vi "MFLI module main.vi"(8 "Update timer[ms]":u32=100, 9 "Master mailbox":T6, 11 "Module mailbox":T6) -> ()   [LabVIEW 2024, in "Lock-in module.lvlib"]
doc: "Module to control MFLI form ZhInst.\nKey typedefs: MFLI_message for module, MFLI_command enum [Initialize, Update, Set module, Set Individual parameters, Set parametres, Get point, Get array, Disconnect, End], MFLI_parameter and value{MFLI_node, value}"
uses:
  Lock-in module.lvlib
  Messenger service/Data types/Mailbox address.ctl
  ctl/ACQ status.ctl
  <instrlib>/Zurich Instruments LabOne/Public/ziTypeHandle.ctl
  <instrlib>/Zurich Instruments LabOne/Public/Modules/ziTypeModHandle.ctl
  ctl/ACQ info.ctl
  ctl/Mode.ctl
  Messenger service/Data types/Module name.ctl
  ctl/MFLI_message for module.ctl
  ctl/MFLI_command enum.ctl
  ctl/MFLI parameters.ctl
  <instrlib>/Zurich Instruments LabOne/Public/Modules/ziTypeModEnum.ctl
  ctl/MFLI_parameter and value.ctl
  ctl/MFLI_node.ctl
  <instrlib>/Zurich Instruments LabOne/Public/Configure/ziSetValueDoubleArray.vi
  <instrlib>/Zurich Instruments LabOne/Public/Configure/ziSetValueDouble.vi
  <instrlib>/Zurich Instruments LabOne/Zurich Instruments LabOne.lvlib
  Messenger service/MessengerLib.lvlib
panel:
  out "error IO":errorcluster
  out "Modulation amplitude [A]":dbl
  out "Multimeter name":string
  out "Multimeter port":refnum<visa-resource-name>
  out "Mode":T1=enum."Point"
  out "ACQ  status":T2={"Lock-in Handle"={"handleValid"=FALSE, "Conn"=0, "Path Prefix"="", "Handle"=0, "Connected"=FALSE, "Clockbase(s)"=0.0}, "Address"="DEV", "ModuleHandles"=[], "Lock-in info"={"In50"=FALSE, "InAC"=FALSE, "InDiff"=FALSE, "Out50"=FALSE, "OutEN"=FALSE, "OutF[Hz]"=0.0, "OutA[V]"=0.0, "DemEN"=FALSE, "Const[ms]"=0.0, "Order[-]"=0, "Phase [°]"=0.0}} {"ModuleHandles"."ModHandle" format="0x%08x"; "ModuleHandles"."Conn" format="0x%08x"; "Lock-in Handle"."Handle" format="0x%08x"; "Lock-in Handle"."Conn" format="0x%08x"}
  out "Selected Device":string
  out "Ended":bool
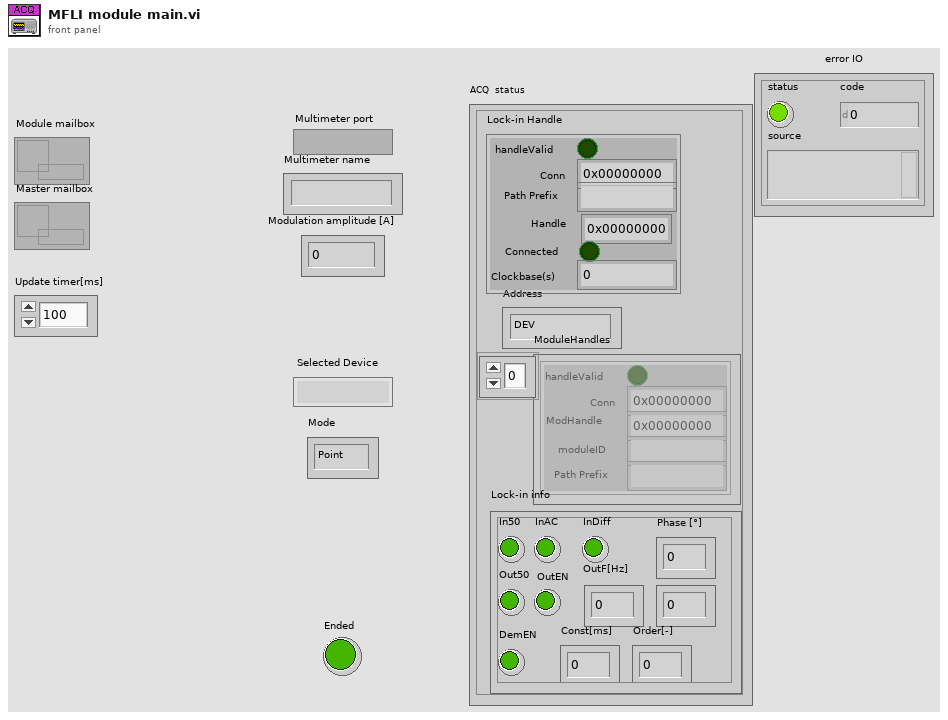
[diagram p1: front panel]
types:
  T1 = typedef "Lock-in module.lvlib/Mode.ctl" = enum16{"None", "Point", "Scope", "Both", "DAQ"}
  T2 = typedef "Lock-in module.lvlib/ACQ status.ctl" = cluster{"Lock-in Handle":T3, "Address":string, "ModuleHandles":T4[], "Lock-in info":T5}
  T3 = typedef "Zurich Instruments LabOne.lvlib/ziTypeHandle.ctl" = cluster{"handleValid":bool, "Conn":u64, "Path Prefix":string, "Handle":u64, "Connected":bool, "Clockbase(s)":dbl}
  T4 = typedef "Zurich Instruments LabOne.lvlib/ziTypeModHandle.ctl" = cluster{"handleValid":bool, "Conn":u64, "ModHandle":u64, "moduleID":string, "Path Prefix":string}
  T5 = typedef "Lock-in module.lvlib/ACQ info.ctl" = cluster{"In50":bool, "InAC":bool, "InDiff":bool, "Out50":bool, "OutEN":bool, "OutF[Hz]":dbl, "OutA[V]":dbl, "DemEN":bool, "Const[ms]":dbl, "Order[-]":i32, "Phase [°]":dbl}
  T6 = typedef "MessengerLib.lvlib/Mailbox address.ctl" = refnum<queue>
  T7 = typedef "Lock-in module.lvlib/MFLI_message for module.ctl" = cluster{"Command":T8, "Data":variant}
  T8 = typedef "Lock-in module.lvlib/MFLI_command enum.ctl" = enum16{"Initialize", "Update", "Set parameters", "Set module", "Set individual parameters", "Get point", "Get array", "Disconnect", "End", "Ignore"}
  T9 = typedef "Module name.ctl" = enum16{"Emty", "Magnet", "VTI", "Excitation", "Servo", "Acquisition", "Rotator", "Digitizer", "SMU2450", "Carousel", "Multimeter", "Tmp monitor", "Power monitor"}
  T10 = typedef "Lock-in module.lvlib/MFLI parameters.ctl" = cluster{"Filter order":dbl, "Filter tau [ms]":dbl, "F_Mod [kHz]":dbl, "Amp_Mod [mV]":dbl, "Enable output":u16, "Phase [°]":dbl}
  T11 = typedef "Lock-in module.lvlib/MFLI_parameter and value.ctl" = cluster{"parameter":T12, "value":dbl}
  T12 = typedef "Lock-in module.lvlib/MFLI_node.ctl" = enum16{"None", "filter_order [-]", "filter_constant [ms]", "in_diff", "in_autorange", "in_imp50", "in_AC", "osc_freq [kHz]", "out_ampl [V]", "out_autorange", "out_imp50", "enable output", "enamble ampl", "scope_enable", "scope_rate", "scope_len", "scope_trigEn", "AuxOut_amplify", "Phase_deg", "AuxOut_select"}
  T13 = typedef "Zurich Instruments LabOne.lvlib/ziTypeModEnum.ctl" = u16
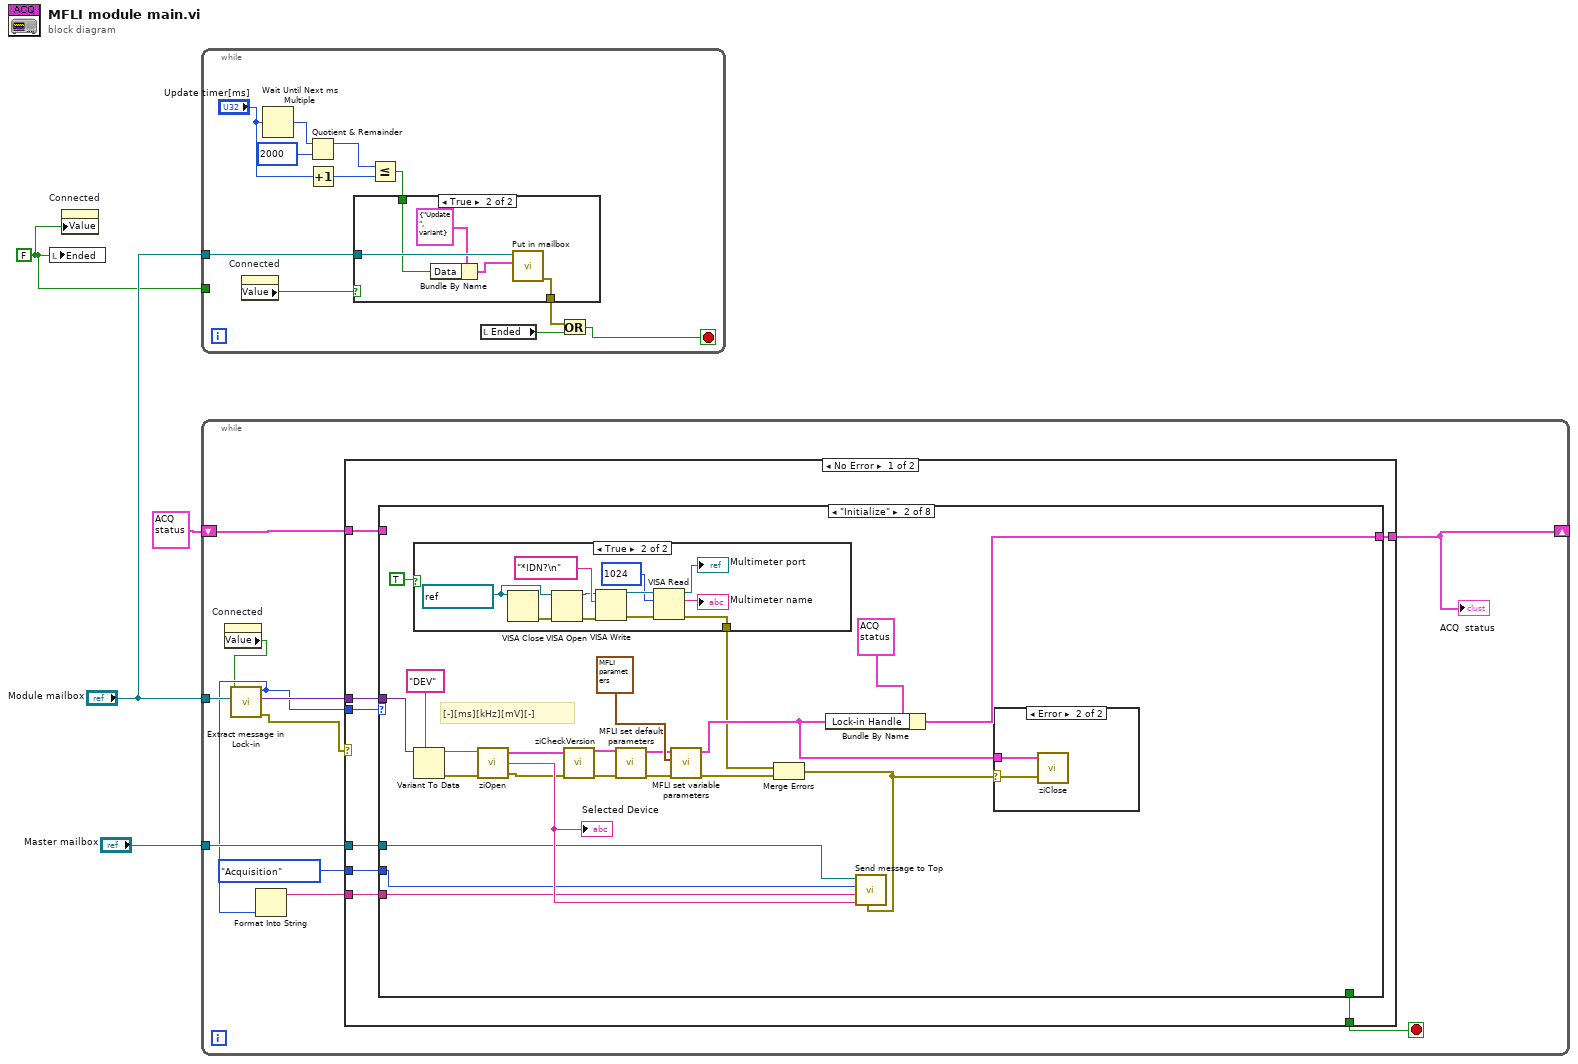
[diagram p0: block diagram]
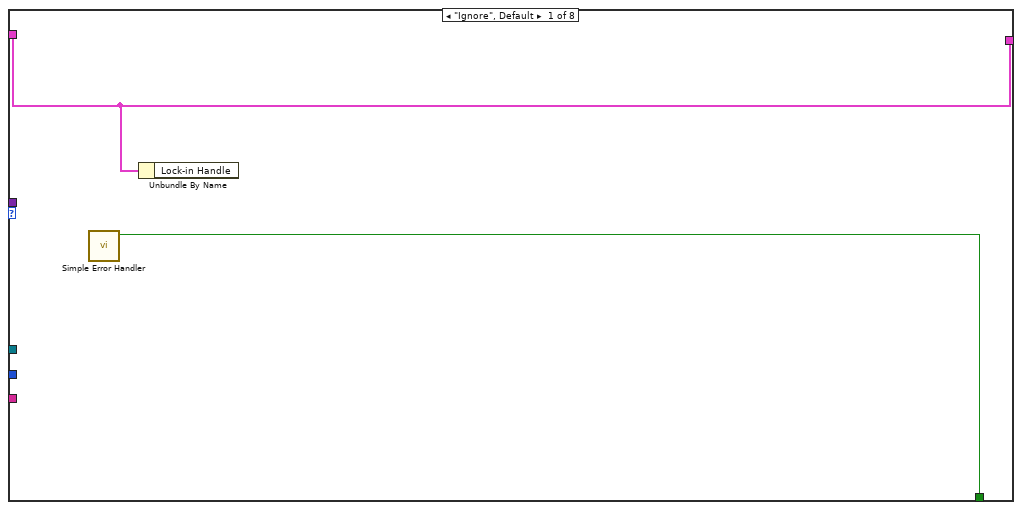
[diagram p2: hidden frame]
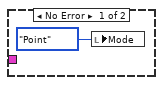
[diagram p4: hidden frame]
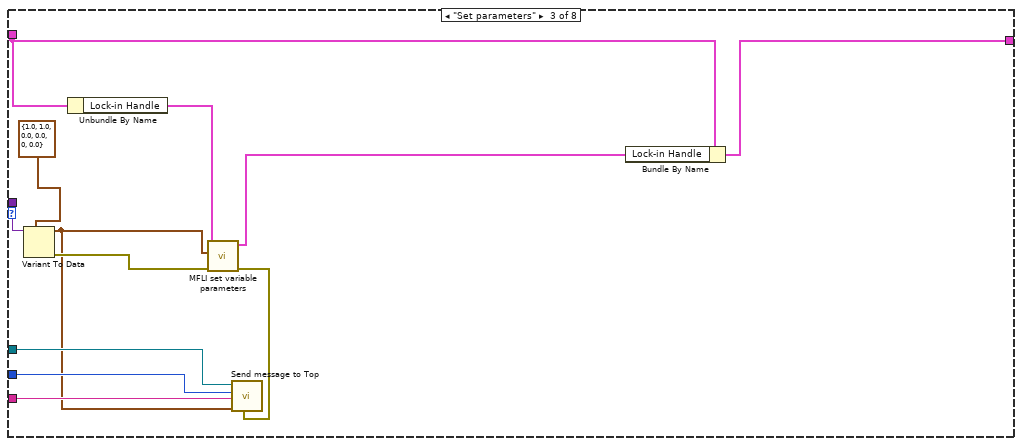
[diagram p5: hidden frame]
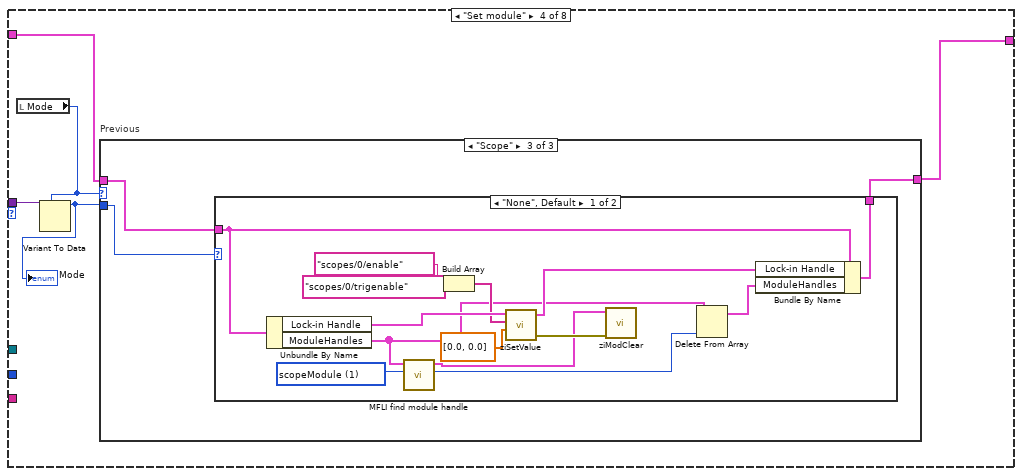
[diagram p6: hidden frame]
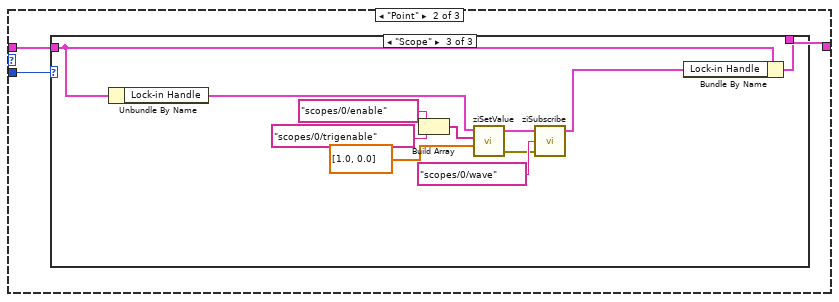
[diagram p8: hidden frame]
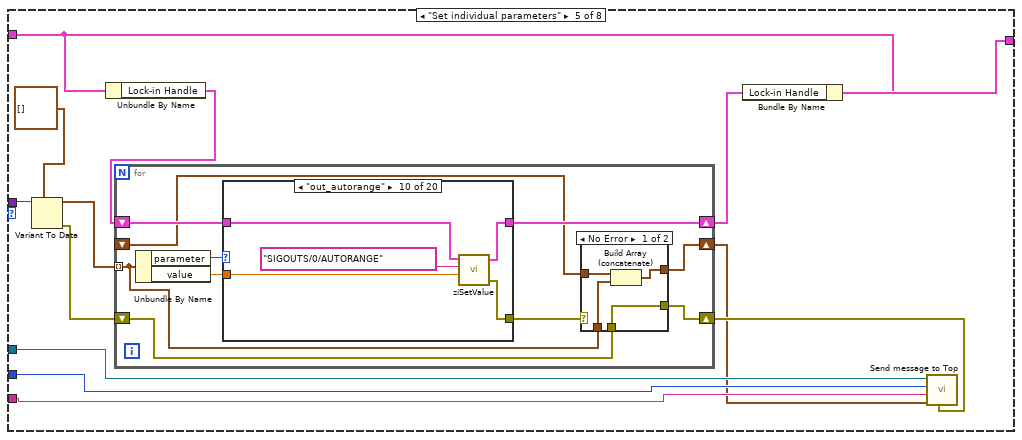
[diagram p12: hidden frame]
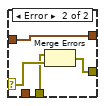
[diagram p13: hidden frame]
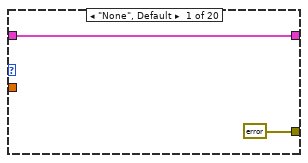
[diagram p14: hidden frame]
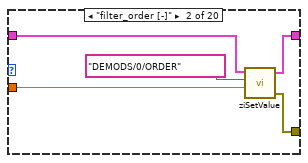
[diagram p15: hidden frame]
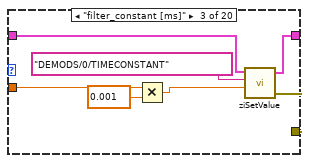
[diagram p16: hidden frame]
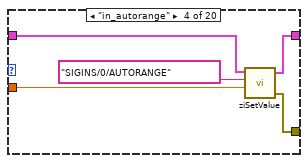
[diagram p17: hidden frame]
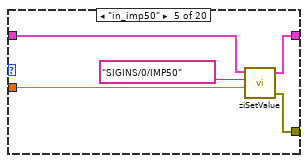
[diagram p18: hidden frame]
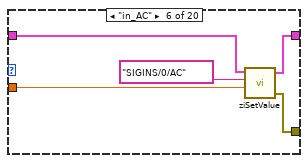
[diagram p19: hidden frame]
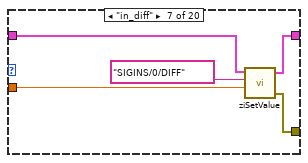
[diagram p20: hidden frame]
diagram:
  w1 = FALSE ("Initialized")
  n1 = local write "Ended"(w1) -> ()
  n2 = property on="Connected" class="Bool (strict)"("Value"=w1) -> ()  [unwired: 2 in, 2 out]
  n3 = while {
    tunnel: "Module mailbox" -> [w15]
    tunnel: w1 -> [_]
    stop <- w6 stop-if-true
    n4 = property on="Connected" class="Bool (strict)"() -> ("Value"=w8:bool)  [unwired: 2 in, 2 out]
    n5 = Wait Until Next ms Multiple(millisecond multiple="Update timer[ms]") -> (millisecond timer value=w14:u32)
    n6 = Quotient & Remainder(x=w14, y=u32 2000) -> (x-y*floor(x/y)=w12:u32)  [unwired: 1 out]
    n7 = Increment(x="Update timer[ms]") -> (x+1=w9:u32)
    n8 = Less Or Equal?(x=w12, y=w9) -> (x <= y?=w10:bool)
    n9 = case shown="True" w8 {
      tunnel: w15 -> [_ w20]
      tunnel: w10 -> [_ w17]
      tunnel: [_ w16] -> w7
      frame False {
      }
      frame True {
        n10 = Bundle By Name(cluster=T7 {"Command"=enum."Update", "Data"=variant} ("MSG for  ACQ"), "Data"=w17) -> (w18:T7)
        n11 = call "Put in mailbox.vi"("Message"=w18, "Queue in"=w20) -> ("error out"=w16:errorcluster)  [unwired: 7 in, 2 out]
      }
    }
    n12 = local read "Ended"() -> (w5:bool)
    n13 = Or(x=w7, y=w5) -> (x .or. y?=w6:bool)
  }
  n14 = while {
    tunnel: "Module mailbox" -> [w31]
    tunnel: "Master mailbox" -> [w30]
    shift-right: [w24] -> _
    shift-left: T2 {"Lock-in Handle"={"handleValid"=FALSE, "Conn"=0, "Path Prefix"="", "Handle"=0, "Connected"=FALSE, "Clockbase(s)"=0.0}, "Address"="DEV", "ModuleHandles"=[], "Lock-in info"={"In50"=FALSE, "InAC"=FALSE, "InDiff"=FALSE, "Out50"=FALSE, "OutEN"=FALSE, "OutF[Hz]"=0.0, "OutA[V]"=0.0, "DemEN"=FALSE, "Const[ms]"=0.0, "Order[-]"=0, "Phase [°]"=0.0}} -> [w28]
    stop <- w23 stop-if-true
    n15 = property on="Connected" class="Bool (strict)"() -> ("Value"=w22:bool)  [unwired: 2 in, 2 out]
    n16 = call "Extract message in Lock-in.vi"("Module mailbox"=w31, "Initialized?"=w22) -> ("error out"=w21:errorcluster, "Data"=w29:variant, "Command out"=w25:T8)  [unwired: 7 in]
    n17 = Format Into String(w25) -> (resulting string=w27:string)  [unwired: 3 in, 1 out]
    n18 = case shown="No Error" w21 {
      selector: w21 -> [_ w345]
      tunnel: w30 -> [w39 _]
      tunnel: w29 -> [w38 _]
      tunnel: w28 -> [w37 w344]
      tunnel: w27 -> [w36 _]
      tunnel: Module_name."Acquisition" ("Module") -> [w35 _]
      tunnel: w25 -> [w34 _]
      tunnel: [w33 w344] -> w24
      tunnel: [w32 w346] -> w23
      frame No Error {
        n19 = case shown="\"Initialize\"" w34 {
          tunnel: w39 -> [_ w57 w85 _ w133 w278 w319 w336]
          tunnel: w38 -> [_ w63 w89 w94 w142 w273 _ _]
          tunnel: [w41 _ _ _ _ _ w310 FALSE] -> w32
          tunnel: [w40 w56 w86 w91 w140 w280 w312 w328] -> w33
          tunnel: w37 -> [w40 _ w87 w90 w138 w277 w320 w337]
          tunnel: w36 -> [_ w53 w84 _ w135 w276 w317 w333]
          tunnel: w35 -> [_ w52 w83 _ w134 w265 w318 w334]
          frame "Ignore", Default {
            n20 = call <vilib>:"Simple Error Handler.vi"() -> ("error?"=w41:bool)  [unwired: 5 in, 4 out]
            n21 = Unbundle By Name(w40) -> ()  [unwired: 1 out]
          }
          frame "Initialize" {
            # "[-][ms][kHz][mV][-]"
            n22 = case shown="True" TRUE {
              tunnel: [_ w66] -> w43
              frame False {
              }
              frame True {
                w73 = refnum<visa-resource-name> "COM6" ("VISA resource name")
                n23 = VISA Close(VISA resource name=w73) -> (error out=w74:errorcluster)  [unwired: 1 in]
                n24 = VISA Open(error in (no error)=w74, VISA resource name=w73) -> (VISA resource name=w68:refnum<visa-resource-name>, error out=w67:errorcluster)  [unwired: 3 in]
                n25 = VISA Write(VISA resource name=w68, write buffer="*IDN?\n", error in (no error)=w67) -> (VISA resource name out=w72:refnum<visa-resource-name>, error out=w71:errorcluster)  [unwired: 1 out]
                n26 = VISA Read(VISA resource name=w72, byte count=u32 1024, error in (no error)=w71) -> (VISA resource name out=→"Multimeter port":refnum<visa-resource-name>, read buffer=→"Multimeter name":string, error out=w66:errorcluster)  [unwired: 1 out]
              }
            }
            n27 = Variant To Data(type="DEV" ("Address"), Variant=w63) -> (data=w61:string, error out=w60:errorcluster)  [unwired: 1 in]
            n28 = call <instrlib>:"ziOpen.vi"("Error In"=w60, "Address"=w61) -> ("Error Out"=w54:errorcluster, "Selected Device"=w58:string, "HandleOut"=w55:T3)  [unwired: 2 in]
            "Selected Device" <- w58
            n29 = call <instrlib>:"ziCheckVersion.vi"("Handle In"=w55, "Error In"=w54) -> ("Handle Out"=w50:T3, "Error Out"=w51:errorcluster)  [unwired: 11 in, 1 out]
            n30 = call "MFLI set default parameters.vi"("error in (no error)"=w51, "Lock-in Handle"=w50) -> ("Error Out"=w47:errorcluster, "Handle Out"=w48:T3)  [unwired: 8 in]
            n31 = call "MFLI set variable parameters.vi"("error in"=w47, "ACQ parameters"=T10 {"Filter order"=5.0, "Filter tau [ms]"=50.0, "F_Mod [kHz]"=10.0, "Amp_Mod [mV]"=100.0, "Enable output"=0, "Phase [°]"=0.0}, "handle in"=w48) -> ("Error Out"=w46:errorcluster, "Handle Out"=w44:T3)  [unwired: 7 in]
            n32 = Merge Errors(w43, w46) -> (w45:errorcluster)
            n33 = Bundle By Name(cluster=T2 {"Lock-in Handle"={"handleValid"=FALSE, "Conn"=0, "Path Prefix"="", "Handle"=0, "Connected"=FALSE, "Clockbase(s)"=0.0}, "Address"="DEV", "ModuleHandles"=[], "Lock-in info"={"In50"=FALSE, "InAC"=FALSE, "InDiff"=FALSE, "Out50"=FALSE, "OutEN"=FALSE, "OutF[Hz]"=0.0, "OutA[V]"=0.0, "DemEN"=FALSE, "Const[ms]"=0.0, "Order[-]"=0, "Phase [°]"=0.0}}, "Lock-in Handle"=w44) -> (w56:T2)
            n34 = call "Send message to Top.vi"("Error in (no error)"=w45, "Data"=w58, "Response"=w53, "Module"=w52, "Mailbox address in"=w57) -> ()  [unwired: 5 in, 2 out]
            n35 = case shown="Error" w45 {
              selector: w45 -> [_ w77]
              tunnel: w44 -> [_ w76]
              frame No Error {
                n36 = local write "Mode"(Mode."Point" ("Mode")) -> ()
              }
              frame Error {
                n37 = call <instrlib>:"ziClose.vi"("Error In"=w77, "Handle In"=w76) -> ()  [unwired: 2 in, 2 out]
              }
            }
          }
          frame "Set parameters" {
            n38 = Variant To Data(type=T10 {"Filter order"=1.0, "Filter tau [ms]"=1.0, "F_Mod [kHz]"=0.0, "Amp_Mod [mV]"=0.0, "Enable output"=0, "Phase [°]"=0.0} ("ACQ parameters"), Variant=w89) -> (data=w78:T10, error out=w80:errorcluster)  [unwired: 1 in]
            n39 = Unbundle By Name(w87) -> ("Lock-in Handle"=w81:T3)
            n40 = call "MFLI set variable parameters.vi"("error in"=w80, "ACQ parameters"=w78, "handle in"=w81) -> ("Error Out"=w82:errorcluster, "Handle Out"=w79:T3)  [unwired: 7 in]
            n41 = call "Send message to Top.vi"("Error in (no error)"=w82, "Data"=w78, "Response"=w84, "Module"=w83, "Mailbox address in"=w85) -> ()  [unwired: 5 in, 2 out]
            n42 = Bundle By Name(cluster=w87, "Lock-in Handle"=w79) -> (w86:T2)
          }
          frame "Set module" {
            n43 = local read "Mode"() -> (w93:T1)
            n44 = Variant To Data(type=w93, Variant=w94) -> (data=w92:T1)  [unwired: 1 in, 1 out]
            "Mode" <- w92
            n45 = case "Previous" shown="\"Scope\"" w93 {
              tunnel: w92 -> [_ w98 w114]
              tunnel: w90 -> [w95 w97 w113]
              tunnel: [w95 w96 w112] -> w91
              frame "None", Default {
              }
              frame "Point" {
                n46 = case shown="\"Scope\"" w98 {
                  tunnel: w97 -> [w99 w100 w110]
                  tunnel: [w99 w100 w111] -> w96
                  frame "None", Default {
                  }
                  frame "Point" {
                  }
                  frame "Scope" {
                    n47 = Unbundle By Name(w110) -> ("Lock-in Handle"=w101:T3)
                    n48 = Build Array("scopes/0/enable", "scopes/0/trigenable") -> (w107:string[])
                    n49 = call-poly <instrlib>:"ziSetValue.vi"("Values"=dbl[] [1.0, 0.0] ("Value"), "Paths"=w107, "Handle In"=w101) -> ("Error Out"=w102:errorcluster, "Handle Out"=w104:T3)  [unwired: 2 in]
                    n50 = call <instrlib>:"ziSubscribe.vi"("error in"=w102, "Path ()"="scopes/0/wave" ("Path"), "Handle In"=w104) -> ("Handle Out"=w103:T3)  [unwired: 1 in, 1 out]
                    n51 = Bundle By Name(cluster=w110, "Lock-in Handle"=w103) -> (w111:T2)
                  }
                }
              }
              frame "Scope" {
                n52 = case shown="\"None\", Default" w114 {
                  tunnel: [w128 w129] -> w112
                  tunnel: w113 -> [w119 w129]
                  frame "None", Default {
                    w120 = T13 1 items=["sweep", "scopeModule", "dataAcquisitionModule", "pidAdvisor", "awgModule", "impedanceModule", "multiDeviceSyncModule", "zoomFFT", "trigger", "deviceSettings", "record"] ("module Id")
                    n53 = Unbundle By Name(w119) -> ("Lock-in Handle"=w125:T3, "ModuleHandles"=w116:T4[])
                    n54 = call "MFLI find module handle.vi"("module Id"=w120, "ModuleHandles"=w116) -> ("index"=w117:i32, "ziModHandle out"=w118:T4)  [unwired: 7 in, 1 out]
                    n55 = Build Array("scopes/0/enable", "scopes/0/trigenable") -> (w122:string[])
                    n56 = call-poly <instrlib>:"ziSetValue.vi"("Values"=dbl[] [0.0, 0.0] ("Value"), "Paths"=w122, "Handle In"=w125) -> ("Error Out"=w123:errorcluster, "Handle Out"=w124:T3)  [unwired: 2 in]
                    n57 = call <instrlib>:"ziModClear.vi"("Error In"=w123, "ziModHandle In"=w118) -> ()  [unwired: 7 in, 2 out]
                    n58 = Delete From Array(array=w116, index=w117) -> (array with subset deleted=w115:T4[])  [unwired: 1 in, 1 out]
                    n59 = Bundle By Name(cluster=w119, "Lock-in Handle"=w124, "ModuleHandles"=w115) -> (w128:T2)
                  }
                  frame "Scope" {
                  }
                }
              }
            }
          }
          frame "Set individual parameters" {
            n60 = Variant To Data(type=T11[] [] ("Array"), Variant=w142) -> (data=w136:T11[], error out=w131:errorcluster)  [unwired: 1 in]
            n61 = Unbundle By Name(w138) -> ("Lock-in Handle"=w139:T3)
            n62 = for {
              tunnel: w136 -> [w145] mode=indexing
              shift-right: [w151] -> w137
              shift-left: w139 -> [w152]
              shift-right: [w147] -> w132
              shift-left: w131 -> [w146]
              shift-right: [w144] -> w130
              shift-left: _ -> [w143]
              n63 = Unbundle By Name(w145) -> ("parameter"=w149:T12, "value"=w150:dbl)
              n64 = case shown="\"out_autorange\"" w149 {
                tunnel: w152 -> [w162 w167 w174 w179 w184 w189 w194 w201 w206 w211 w216 w221 w226 w231 w234 w241 w244 w249 w254 w259]
                tunnel: [w162 w166 w173 w178 w183 w188 w193 w200 w205 w210 w215 w220 w225 w230 w235 w240 w245 w250 w255 w260] -> w151
                tunnel: w150 -> [_ w165 w172 w177 w182 w187 w192 w197 w204 w209 w214 w219 w224 w228 w233 w239 w243 w248 w253 w258]
                tunnel: [errorcluster {"status"=FALSE, "code"=0, "source"=""} ("Error Out") w163 w170 w175 w180 w185 w190 w199 w202 w207 w212 w217 w222 w229 w236 w237 w246 w251 w256 w261] -> w148
                frame "None", Default {
                }
                frame "filter_order [-]" {
                  n65 = call-poly <instrlib>:"ziSetValue.vi"("Value"=w165, "Path"="DEMODS/0/ORDER", "Handle In"=w167) -> ("Error Out"=w163:errorcluster, "Handle Out"=w166:T3)  [unwired: 2 in]
                }
                frame "filter_constant [ms]" {
                  n66 = Multiply(x=w172, y=0.001) -> (x*y=w169:dbl)
                  n67 = call-poly <instrlib>:"ziSetValue.vi"("Value"=w169, "Path"="DEMODS/0/TIMECONSTANT", "Handle In"=w174) -> ("Error Out"=w170:errorcluster, "Handle Out"=w173:T3)  [unwired: 2 in]
                }
                frame "in_autorange" {
                  n68 = call-poly <instrlib>:"ziSetValue.vi"("Value"=w177, "Path"="SIGINS/0/AUTORANGE", "Handle In"=w179) -> ("Error Out"=w175:errorcluster, "Handle Out"=w178:T3)  [unwired: 2 in]
                }
                frame "in_imp50" {
                  n69 = call-poly <instrlib>:"ziSetValue.vi"("Value"=w182, "Path"="SIGINS/0/IMP50", "Handle In"=w184) -> ("Error Out"=w180:errorcluster, "Handle Out"=w183:T3)  [unwired: 2 in]
                }
                frame "in_AC" {
                  n70 = call-poly <instrlib>:"ziSetValue.vi"("Value"=w187, "Path"="SIGINS/0/AC", "Handle In"=w189) -> ("Error Out"=w185:errorcluster, "Handle Out"=w188:T3)  [unwired: 2 in]
                }
                frame "in_diff" {
                  n71 = call-poly <instrlib>:"ziSetValue.vi"("Value"=w192, "Path"="SIGINS/0/DIFF", "Handle In"=w194) -> ("Error Out"=w190:errorcluster, "Handle Out"=w193:T3)  [unwired: 2 in]
                }
                frame "osc_freq [kHz]" {
                  n72 = Multiply(x=w197, y=1000.0) -> (x*y=w196:dbl)
                  n73 = call-poly <instrlib>:"ziSetValue.vi"("Value"=w196, "Path"="OSCS/0/FREQ", "Handle In"=w201) -> ("Error Out"=w199:errorcluster, "Handle Out"=w200:T3)  [unwired: 2 in]
                }
                frame "out_ampl [V]" {
                  n74 = call-poly <instrlib>:"ziSetValue.vi"("Value"=w204, "Path"="SIGOUTS/0/AMPLITUDES/1", "Handle In"=w206) -> ("Error Out"=w202:errorcluster, "Handle Out"=w205:T3)  [unwired: 2 in]
                }
                frame "out_autorange" {
                  n75 = call-poly <instrlib>:"ziSetValue.vi"("Value"=w209, "Path"="SIGOUTS/0/AUTORANGE", "Handle In"=w211) -> ("Error Out"=w207:errorcluster, "Handle Out"=w210:T3)  [unwired: 2 in]
                }
                frame "out_imp50" {
                  n76 = call-poly <instrlib>:"ziSetValue.vi"("Value"=w214, "Path"="SIGOUTS/0/IMP50", "Handle In"=w216) -> ("Error Out"=w212:errorcluster, "Handle Out"=w215:T3)  [unwired: 2 in]
                }
                frame "enable output" {
                  n77 = call-poly <instrlib>:"ziSetValue.vi"("Value"=w219, "Path"="SIGOUTS/0/ON", "Handle In"=w221) -> ("Error Out"=w217:errorcluster, "Handle Out"=w220:T3)  [unwired: 2 in]
                }
                frame "enamble ampl" {
                  n78 = call-poly <instrlib>:"ziSetValue.vi"("Value"=w224, "Path"="SIGOUTS/0/ENABLES/1", "Handle In"=w226) -> ("Error Out"=w222:errorcluster, "Handle Out"=w225:T3)  [unwired: 2 in]
                }
                frame "scope_enable" {
                  n79 = call-poly <instrlib>:"ziSetValue.vi"("Value"=w228, "Path"="scopes/0/enable", "Handle In"=w231) -> ("Error Out"=w229:errorcluster, "Handle Out"=w230:T3)  [unwired: 2 in]
                }
                frame "scope_rate" {
                  n80 = call-poly <instrlib>:"ziSetValue.vi"("Value"=w233, "Path"="scopes/0/time", "Handle In"=w234) -> ("Error Out"=w236:errorcluster, "Handle Out"=w235:T3)  [unwired: 2 in]
                }
                frame "scope_trigEn" {
                  n81 = call-poly <instrlib>:"ziSetValue.vi"("Value"=w239, "Path"="SCOPES/0/TRIGENABLE", "Handle In"=w241) -> ("Error Out"=w237:errorcluster, "Handle Out"=w240:T3)  [unwired: 2 in]
                }
                frame "scope_len" {
                  n82 = call-poly <instrlib>:"ziSetValue.vi"("Value"=w243, "Path"="scopes/0/length", "Handle In"=w244) -> ("Error Out"=w246:errorcluster, "Handle Out"=w245:T3)  [unwired: 2 in]
                }
                frame "AuxOut_amplify" {
                  n83 = call-poly <instrlib>:"ziSetValue.vi"("Value"=w248, "Path"="auxouts/0/scale", "Handle In"=w249) -> ("Error Out"=w251:errorcluster, "Handle Out"=w250:T3)  [unwired: 2 in]
                }
                frame "Phase_deg" {
                  n84 = call-poly <instrlib>:"ziSetValue.vi"("Value"=w253, "Path"="demods/1/phaseshift", "Handle In"=w254) -> ("Error Out"=w256:errorcluster, "Handle Out"=w255:T3)  [unwired: 2 in]
                }
                frame "AuxOut_select" {
                  n85 = call-poly <instrlib>:"ziSetValue.vi"("Value"=w258, "Path"="auxouts/0/outputselect", "Handle In"=w259) -> ("Error Out"=w261:errorcluster, "Handle Out"=w260:T3)  [unwired: 2 in]
                }
              }
              n86 = case shown="No Error" w148 {
                selector: w148 -> [_ w160]
                tunnel: [w156 w159] -> w147
                tunnel: w146 -> [w156 w158]
                tunnel: w145 -> [w154 _]
                tunnel: [w155 w157] -> w144
                tunnel: w143 -> [w153 w157]
                frame No Error {
                  n87 = Build Array (concatenate)(w153, w154) -> (w155:T11[])
                }
                frame Error {
                  n88 = Merge Errors(w158, w160) -> (w159:errorcluster)
                }
              }
            }
            n89 = Bundle By Name(cluster=w138, "Lock-in Handle"=w137) -> (w140:T2)
            n90 = call "Send message to Top.vi"("Error in (no error)"=w132, "Data"=w130, "Response"=w135, "Module"=w134, "Mailbox address in"=w133) -> ()  [unwired: 5 in, 2 out]
          }
          frame "Update" {
            n91 = Unbundle By Name(w277) -> ("Lock-in info"=w270:T5, "ModuleHandles"=w267:T4[], "Lock-in Handle"=w279:T3)
            n92 = Variant To Data(type=TRUE, Variant=w273) -> (data=w271:bool, error out=w274:errorcluster)  [unwired: 1 in]
            n93 = case shown="True" w271 {
              tunnel: w279 -> [w284 w294]
              tunnel: [w284 w293] -> w266
              tunnel: w278 -> [w281 w292]
              tunnel: [w282 w290] -> w264
              tunnel: w265 -> [_ w289]
              tunnel: [w281 w288] -> w269
              tunnel: w276 -> [_ w287]
              tunnel: [w283 w286] -> w275
              tunnel: w274 -> [w282 w285]
              tunnel: w270 -> [w283 _]
              frame False {
              }
              frame True {
                n94 = call "Lock-in update.vi"("error in (no error)"=w285, "Lock-in Handle"=w294) -> ("error out"=w291:errorcluster, "Lock-in info"=w286:T5, "Handle Out"=w293:T3)  [unwired: 7 in]
                n95 = call "Send message to Top.vi"("Error in (no error)"=w291, "Data"=w286, "Response"=w287, "Module"=w289, "Mailbox address in"=w292) -> ("Error out"=w290:errorcluster, "Mailbox address out"=w288:T6)  [unwired: 5 in]
              }
            }
            n96 = case shown="True" w271 {
              tunnel: w265 -> [_ w300]
              tunnel: w269 -> [_ w297]
              frame False {
              }
              frame True {
                n97 = local read "Multimeter port"() -> (w308:refnum<visa-resource-name>)
                n98 = VISA Write(VISA resource name=w308, write buffer="READ?\n") -> (VISA resource name out=w307:refnum<visa-resource-name>, error out=w296:errorcluster)  [unwired: 1 in, 1 out]
                n99 = VISA Read(VISA resource name=w307, byte count=u32 1024, error in (no error)=w296) -> (read buffer=w305:string, error out=w295:errorcluster)  [unwired: 2 out]
                n100 = String Subset(string=w305, length (rest)=11 ("length (rest)")) -> (substring=w306:string)  [unwired: 1 in]
                n101 = Scan Value(string=w306, format string="%g") -> (value=w299:dbl)  [unwired: 1 in, 1 out]
                "Modulation amplitude [A]" <- w299
                n102 = call "Send message to Top.vi"("Error in (no error)"=w295, "Data"=w299, "Response"="Get ModA", "Module"=w300, "Mailbox address in"=w297) -> ()  [unwired: 5 in, 2 out]
              }
            }
            n103 = local read "Mode"() -> (w268:T1)
            n104 = call "MFLI read data.vi"("Module"=w265, "ModuleHandles in"=w267, "error in (no error)"=w264, "lock-in handle in"=w266, "Mode"=w268, "Queue in"=w269) -> ("ModuleHandles out"=w262:T4[], "Handle Out out"=w263:T3)  [unwired: 4 in]
            n105 = Bundle By Name(cluster=w277, "Lock-in Handle"=w263, "ModuleHandles"=w262, "Lock-in info"=w275) -> (w280:T2)
          }
          frame "End" {
            w310 = TRUE
            n106 = Unbundle By Name(w320) -> ("Lock-in Handle"=w314:T3)
            n107 = local read "Mode"() -> (w316:T1)
            n108 = case shown="\"Scope\", \"Both\"" w316 {
              tunnel: w314 -> [w322 w326]
              tunnel: [w322 w324] -> w315
              tunnel: [_ w323] -> w309
              frame "None", Default {
              }
              frame "Scope", "Both" {
                n109 = call <instrlib>:"ziUnSubscribe.vi"("Path (\"/\")"="scopes/0/wave" ("Path"), "Handle in"=w326) -> ("error out"=w323:errorcluster, "Handle out"=w324:T3)  [unwired: 2 in]
              }
            }
            n110 = call <instrlib>:"ziClose.vi"("Error In"=w309, "Handle In"=w315) -> ("Handle Out"=w311:T3)  [unwired: 2 in, 1 out]
            n111 = call "Send message to Top.vi"("Data"=w311, "Response"=w317, "Module"=w318, "Mailbox address in"=w319) -> ()  [unwired: 6 in, 2 out]
            n112 = case shown="False" TRUE {
              frame False {
              }
              frame True {
                n113 = local read "Multimeter port"() -> (w321:refnum<visa-resource-name>)
                n114 = VISA Close(VISA resource name=w321) -> ()  [unwired: 1 in, 1 out]
              }
            }
            n115 = Bundle By Name(cluster=w320, "Lock-in Handle"=w311) -> (w312:T2)
            "Ended" <- w310
          }
          frame "Disconnect" {
            n116 = Unbundle By Name(w337) -> ("Lock-in Handle"=w330:T3)
            n117 = local read "Mode"() -> (w332:T1)
            n118 = case shown="\"Scope\", \"Both\"" w332 {
              tunnel: w330 -> [w340 w343]
              tunnel: [w340 w341] -> w331
              frame "None", Default {
              }
              frame "Scope", "Both" {
                n119 = call <instrlib>:"ziUnSubscribe.vi"("Path (\"/\")"="scopes/0/wave" ("Path"), "Handle in"=w343) -> ("Handle out"=w341:T3)  [unwired: 2 in, 1 out]
              }
            }
            n120 = call <instrlib>:"ziClose.vi"("Handle In"=w331) -> ("Handle Out"=w327:T3)  [unwired: 3 in, 1 out]
            n121 = call "Send message to Top.vi"("Data"=w327, "Response"=w333, "Module"=w334, "Mailbox address in"=w336) -> ()  [unwired: 6 in, 2 out]
            n122 = case shown="True" TRUE {
              frame False {
              }
              frame True {
                n123 = local read "Multimeter port"() -> (w339:refnum<visa-resource-name>)
                n124 = VISA Close(VISA resource name=w339) -> ()  [unwired: 1 in, 1 out]
              }
            }
            n125 = local write "Ended"(FALSE ("Initialized")) -> ()
            n126 = Bundle By Name(cluster=w337, "Lock-in Handle"=w327) -> (w328:T2)
          }
        }
      }
      frame Error {
        w346 = TRUE ("error?")
        n127 = local write "Ended"(w346) -> ()
        "error IO" <- w345
      }
    }
    "ACQ  status" <- w24
  }
